vi "(Var) Get_HVPS_1.vi"() -> ()   [LabVIEW 2017]
panel:
  out "G1. Q Stop":bool=TRUE
  out "G1. Stop":bool=TRUE
  out "G1. Start":bool=TRUE
  out "G1. Error ?":bool
  out "G1. mA":dbl
  out "G1. KV":dbl
  out "G1. Read Mode":string
  out "G1. Read HV":string
  out "G1. Read State":string
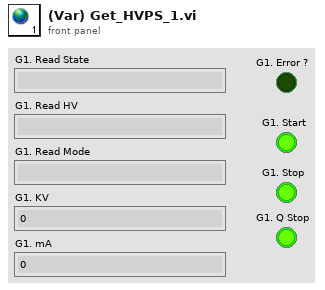
[diagram p1: front panel]
diagram:
